vi "Wave-Write EPL Chunk.vi"(8 "error in (no error)":errorcluster, 10 "EPL Variables":T1[](array[typedef]), 11 "refnum":refnum<file>) -> (0 "error out":errorcluster, 3 "refnum out":refnum<file>)   [LabVIEW 2020]
uses:
  Wave-EPL Chunk Variable.ctl
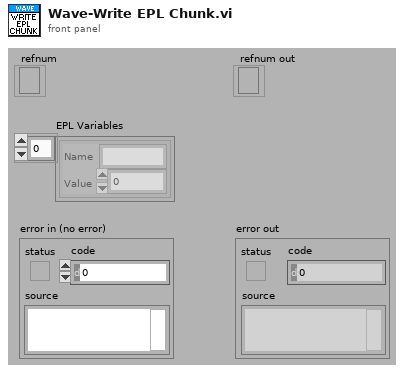
[diagram p1: front panel]
types:
  T1 = typedef "Wave-EPL Chunk Variable.ctl" = cluster{"Name":string, "Value":dbl}
  T2 = enum16{"big-endian, network order", "native, host order", "little-endian"}
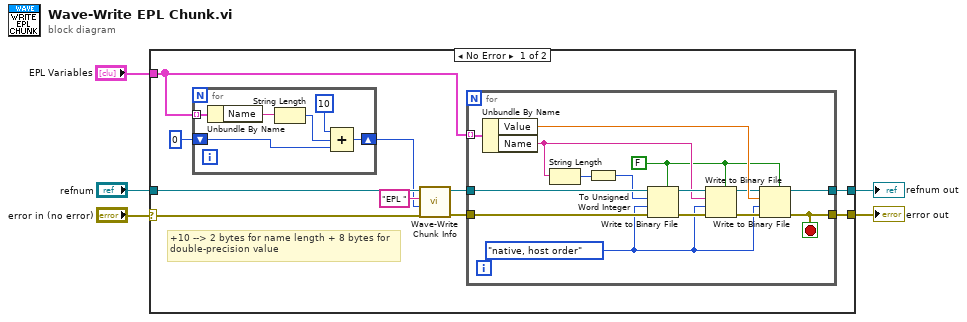
[diagram p0: block diagram]
diagram:
  n1 = case shown="No Error" "error in (no error)" {
    selector: "error in (no error)" -> [w10 w37]
    tunnel: "refnum" -> [w11 w38]
    tunnel: [w15 w38] -> w4
    tunnel: [w14 w37] -> w2
    tunnel: "EPL Variables" -> [w8 _]
    frame No Error {
      # "+10 --> 2 bytes for name length + 8 bytes for double-precision value"
      n2 = for {
        tunnel: w8 -> [w21] mode=indexing
        shift-right: [w16] -> w6
        shift-left: 0 -> [w17]
        n3 = Unbundle By Name(w21) -> ("Name"=w20:string)
        n4 = String Length(string=w20) -> (length=w19:i32)
        n5 = Compound Arithmetic op=ADD(10 ("value"), w19, w17) -> (w16:i32)
      }
      n6 = call "Wave-Write Chunk Info.vi"("error in (no error)"=w10, "Size"=w6, "ID"="EPL ", "refnum"=w11) -> ("error out"=w13:errorcluster, "refnum out"=w12:refnum<file>)  [unwired: 6 in]
      n7 = for {
        tunnel: w12 -> [w33]
        tunnel: w13 -> [w34]
        tunnel: w8 -> [w36] mode=indexing
        tunnel: [w25] -> w15
        tunnel: [w24] -> w14
        stop <- w24 stop-if-true
        w23 = FALSE ("prepend array or string size? (T)")
        w22 = T2."native, host order" ("byte order (0:big-endian, network order)")
        n8 = Unbundle By Name(w36) -> ("Value"=w27:dbl, "Name"=w29:string)
        n9 = String Length(string=w29) -> (length=w35:i32)
        n10 = To Unsigned Word Integer(number=w35) -> (unsigned 16bit integer=w32:u16)
        n11 = Write to Binary File(file (use dialog)=w33, data=w32, error in=w34, 5:w23, 9:w22) -> (refnum out=w30:refnum<file>, error out=w31:errorcluster)  [unwired: 1 in, 1 out]
        n12 = Write to Binary File(file (use dialog)=w30, data=w29, error in=w31, 5:w23, 9:w22) -> (refnum out=w26:refnum<file>, error out=w28:errorcluster)  [unwired: 1 in, 1 out]
        n13 = Write to Binary File(file (use dialog)=w26, data=w27, error in=w28, 5:w23, 9:w22) -> (refnum out=w25:refnum<file>, error out=w24:errorcluster)  [unwired: 1 in, 1 out]
      }
    }
    frame Error {
    }
  }
  "error out" <- w2
  "refnum out" <- w4
